vi "begin direct write.vi"(5 "requestID":u32, 7 "event":refnum<user-event>, 8 "error in":errorcluster, 10 "data":string, 11 "socket":u64) -> (0 "error out":errorcluster, 2 "remaining data":string)   [LabVIEW 2016, in "async tls dl.lvlib"]
uses:
  async tls dl.lvlib
  action complete event.ctl
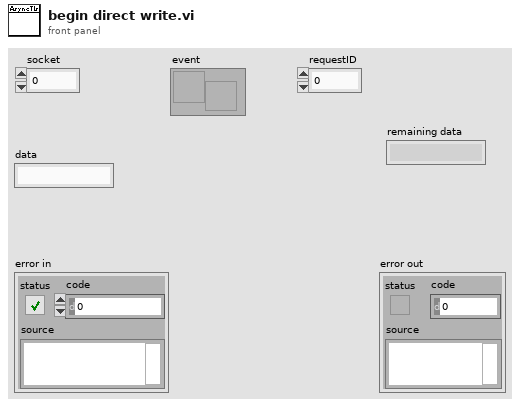
[diagram p1: front panel]
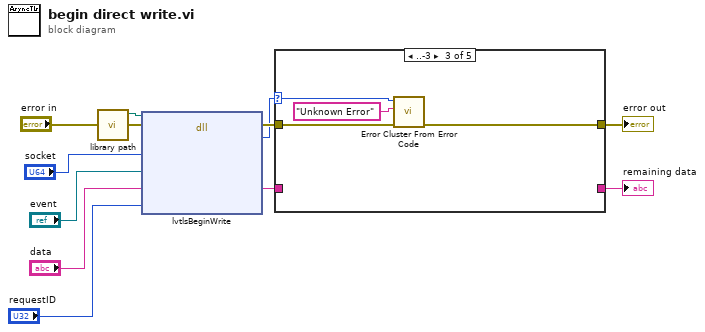
[diagram p0: block diagram]
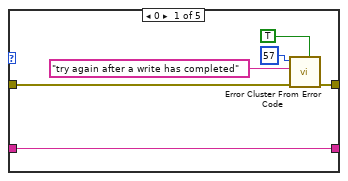
[diagram p2: hidden frame]
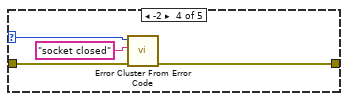
[diagram p4: hidden frame]
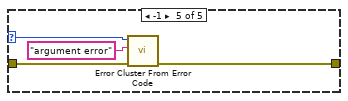
[diagram p5: hidden frame]
diagram:
  n1 = call "library path.vi"() -> ("path"=w4:path)  [unwired: 11 in]
  n2 = dll-call lib="C:/Users/IEUser/Desktop/libasynclvtls/lvasynctls.dll" fn="lvtlsBeginWrite"(path in=w4, error in="error in", "socket"="socket", "event"="event", "data"="data", "requestID"="requestID") -> (error out=w11:errorcluster, "return code"=w10:i64, "data"=w1:string)  [unwired: 4 in, 1 out]
  n3 = case shown="..-3" w10 {
    selector: w10 -> [_ _ w21 w25 w29]
    tunnel: w11 -> [w16 w18 w22 w26 w30]
    tunnel: [w17 w18 w20 w24 w28] -> w9
    tunnel: w1 -> [w15 _ _ _ _]
    tunnel: [w15 _ _ _ _] -> w3
    frame 0 {
      n4 = call <vilib>:"Error Cluster From Error Code.vi"("is warning? (False)"=TRUE, "error in (no error)"=w16, "error message (\"\")"="try again after a write has completed" ("error message (\"\")"), "error code (0)"=57) -> ("error out"=w17:errorcluster)  [unwired: 5 in]
    }
    frame 1.. {
    }
    frame ..-3 {
      n5 = call <vilib>:"Error Cluster From Error Code.vi"("error in (no error)"=w22, "error message (\"\")"="Unknown Error" ("error message (\"\")"), "error code (0)"=w21) -> ("error out"=w20:errorcluster)  [unwired: 6 in]
    }
    frame -2 {
      n6 = call <vilib>:"Error Cluster From Error Code.vi"("error in (no error)"=w26, "error message (\"\")"="socket closed" ("error message (\"\")"), "error code (0)"=w25) -> ("error out"=w24:errorcluster)  [unwired: 6 in]
    }
    frame -1 {
      n7 = call <vilib>:"Error Cluster From Error Code.vi"("error in (no error)"=w30, "error message (\"\")"="argument error" ("error message (\"\")"), "error code (0)"=w29) -> ("error out"=w28:errorcluster)  [unwired: 6 in]
    }
  }
  "error out" <- w9
  "remaining data" <- w3
